vi "FlatToRichcif_manager_PluginTypeReply.vi"(5 "OutputClusterType":T1, 11 "InputCluster":T5) -> (3 "OutputCluster":T1)   [LabVIEW 2021, in "CIF_Manager_client.lvlib"]
uses:
  CIF_Manager_client.lvlib
  cif_manager_PluginTypeReply_Flat.ctl
  cif_manager_PluginType_Flat.ctl
  cif_manager_PluginVersion_Flat.ctl
  cif_manager_Error_Flat.ctl
  cif_manager_PluginTypeReply.ctl
  cif_manager_PluginType.ctl
  cif_manager_PluginVersion.ctl
  cif_manager_Error.ctl
  FlatToRichcif_manager_PluginVersion.vi
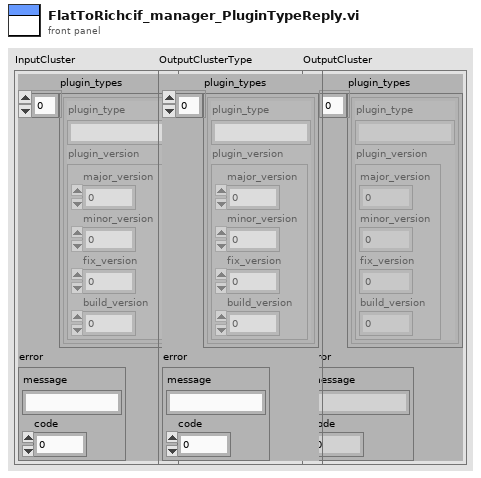
[diagram p1: front panel]
types:
  T1 = typedef "CIF_Manager_client.lvlib/cif_manager_PluginTypeReply.ctl" = cluster{"plugin_types":T2[], "error":T4}
  T2 = typedef "CIF_Manager_client.lvlib/cif_manager_PluginType.ctl" = cluster{"plugin_type":string, "plugin_version":T3}
  T3 = typedef "CIF_Manager_client.lvlib/cif_manager_PluginVersion.ctl" = cluster{"major_version":i32, "minor_version":i32, "fix_version":i32, "build_version":i32}
  T4 = typedef "CIF_Manager_client.lvlib/cif_manager_Error.ctl" = cluster{"message":string, "code":i32}
  T5 = typedef "CIF_Manager_client.lvlib/cif_manager_PluginTypeReply_Flat.ctl" = cluster{"plugin_types":T6[], "error":T8}
  T6 = typedef "CIF_Manager_client.lvlib/cif_manager_PluginType_Flat.ctl" = cluster{"plugin_type":string, "plugin_version":T7}
  T7 = typedef "CIF_Manager_client.lvlib/cif_manager_PluginVersion_Flat.ctl" = cluster{"major_version":i32, "minor_version":i32, "fix_version":i32, "build_version":i32}
  T8 = typedef "CIF_Manager_client.lvlib/cif_manager_Error_Flat.ctl" = cluster{"message":string, "code":i32}
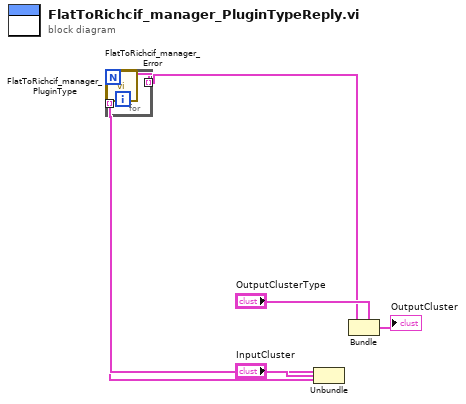
[diagram p0: block diagram]
diagram:
  n1 = Unbundle "Unbundle"("InputCluster") -> ("plugin_types"=w4:T6[], "error"=w2:T8)
  n2 = call "FlatToRichcif_manager_Error.vi"("InputCluster"=w2) -> ("OutputCluster"=w1:T4)  [unwired: 10 in]
  n3 = for {
    tunnel: w4 -> [w9] mode=indexing
    tunnel: [w8] -> w3 mode=indexing
    n4 = call "FlatToRichcif_manager_PluginType.vi"("InputCluster"=w9) -> ("OutputCluster"=w8:T2)  [unwired: 10 in]
  }
  n5 = Bundle "Bundle"(cluster="OutputClusterType", "plugin_types"=w3, "error"=w1) -> (→"OutputCluster":T1)
